vi "FPGA 796xR - Bak20470818.vi"() -> ()   [LabVIEW 2015]
uses:
  Controls/FPGA_Frame State.ctl
  <vilib>/Platform/TimedLoop/XDataNode/timing_clust.ctl
  <vilib>/Platform/TimedLoop/XDataNode/nitl_modes.ctl
  <vilib>/Platform/TimedLoop/XDataNode/wakeup.ctl
  <vilib>/rvi/Emulation/niFpgaSctlEmulationGetInTimedLoop.vi
  <vilib>/rvi/Emulation/niFpgaProcessEmulError.vi
  <vilib>/rvi/Emulation/niFpgaEmulationReportErrorSimple.vi
  <vilib>/rvi/Emulation/niFpgaGetClockAttributes.vi
  <vilib>/rvi/Emulation/niFpgaCriticalErrorInLSC.vi
  <vilib>/rvi/eio/common/nirviEmuTemplateMethod_errors.vi
  <vilib>/rvi/interface/RandomDataEmulation/niFpgaRandomDataHandleErrors.vi
  <vilib>/rvi/Memory/Memory_Emulation/nirvimemoryFastEmulation.vi
  <vilib>/rvi/Memory/Memory_Emulation/nirvimemoryEmulation.vi
  <vilib>/rvi/Emulation/niFpgaEmulationIsFPGAContextNoSignature.vi
  <vilib>/rvi/DataTransferAndStorage/Container/Common/niFpgaContainerGetUniqueNameForEmu.vi
  <vilib>/rvi/errors/nirviReportUnexpectedCaseInternalError (U32).vi
  <vilib>/Platform/TimedLoop/XDataNode/XDataNode.xnode
  <vilib>/eio/EIONode/EIONode.xnode
  <vilib>/rvi/DataTransferAndStorage/Container/XNode/niFpgaContainer.xnode
  <vilib>/rvi/interface/RandomDataEmulation/nirviRandomDataFpgaReadWriteTemplate.vi
  <vilib>/rvi/FXPMathLib/FxpMul/XNode/nifxpmath_Multiplier.xnode
  <vilib>/rvi/FXPMathLib/FxpAdd/XNode/nifxpmath_Add.xnode
  <vilib>/Platform/TimedLoop/XDataNode/XDNodeRunTimeDep.lvlib
  <instrlib>/_niInstr/Basic Elements/v1/FPGA/niInstr Basic Elements v1 FPGA.lvlib
  <vilib>/rvi/FXPMathLib/sim/FxpSim.dll
panel:
  out "Acq. Point Dis.":u16
  in  "Acq.Start":u16
  in  "Acq.Start FXP":fxp<+,16,0>
  out "Acq Pixel Number":u32
  out "AcqPoint 元素数量":u32
  in  "Microscope":enum16{"Miniature", "Benchtop"}(ring)
  out "No Remind":bool
  out "Remind Element":u32
  in  "FOCUS":bool
  out "Wait Frame State":T1
  in  "Line":u16
  in  "Pixel/Line":u16
  out "Adapter Module Present":bool
  out "Adapter Module ID Expected":u32
  out "Adapter Module ID Inserted":u32
  out "Adapter Module Initialization Done":bool
  out "Adapter Module ID Mismatch":bool
  in  "Adapter Module Do User Command Commit":bool caption="(Mech Action: Latch)"
  in  "Adapter Module User Command":u8
  out "Adapter Module User Command Idle":bool
  out "Adapter Module User Command Status":u8
  in  "Adapter Module User Data 0":u8
  in  "Adapter Module User Data 1":u8
  out "Adapter Module PLL Locked":bool
  # "Acquisition Parameters"
  # "Acquisition Control"
  # "User Command Load"
  # "Fpga status"
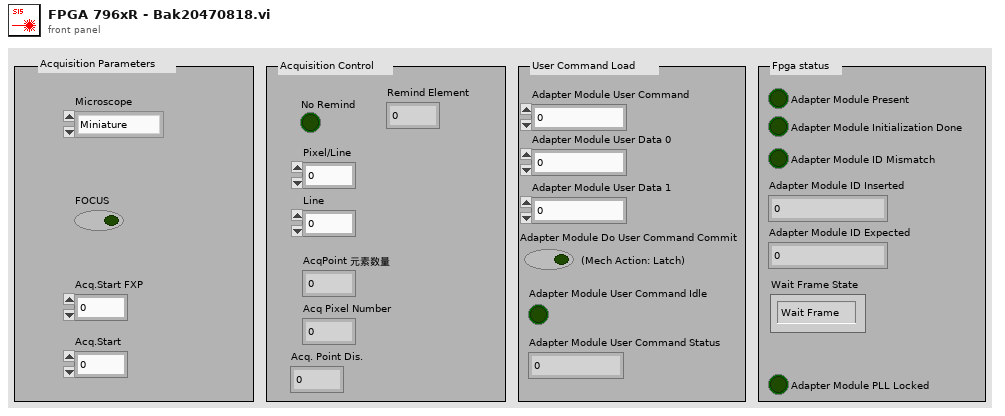
[diagram p1: front panel]
types:
  T1 = typedef "FPGA_Frame State.ctl" = enum16{"Wait Frame", "Start Frame", "Framing"}
  T2 = typedef "XDNodeRunTimeDep.lvlib/timing_clust.ctl" = cluster{"Expected End [f-1]":u64, "Actual End [f-1]":u64, "Finished Late? [f-1]":bool, "Expected End [i-1]":u64, "Actual End [i-1]":u64, "Finished Late? [i-1]":bool, "Expected Start [i]":u64, "Actual Start [i]":u64, "Expected Start [f]":u64, "Actual Start [f]":u64, "Source Name":string, "Structure Name":string, "Period":i64, "Deadline":i64, "Offset":i64, "Start":i64, "Priority":i32, "Timeout":i32, "Mode":T3, "Wakeup Reason":T4, "Error":errorcluster, "Source Type":string, "Secondary Source Type":string, "Global End Time":u64, "Global Start Time":u64, "Frame Duration":u64, "Iteration Duration":u64, "Assigned CPU":i32, "I/O Scan Engine Mode":u32}
  T3 = typedef "XDNodeRunTimeDep.lvlib/nitl_modes.ctl" = enum32{"No Change", "Process missed periods, maintain original phase", "Discard missed periods, maintain original phase", "Process missed periods, ignore original phase", "Discard missed periods, ignore original phase"}
  T4 = typedef "XDNodeRunTimeDep.lvlib/wakeup.ctl" = enum32{"Normal", "Aborted", "Asynchronous wakeup", "Timing source error", "Timed loop error", "Timeout"}
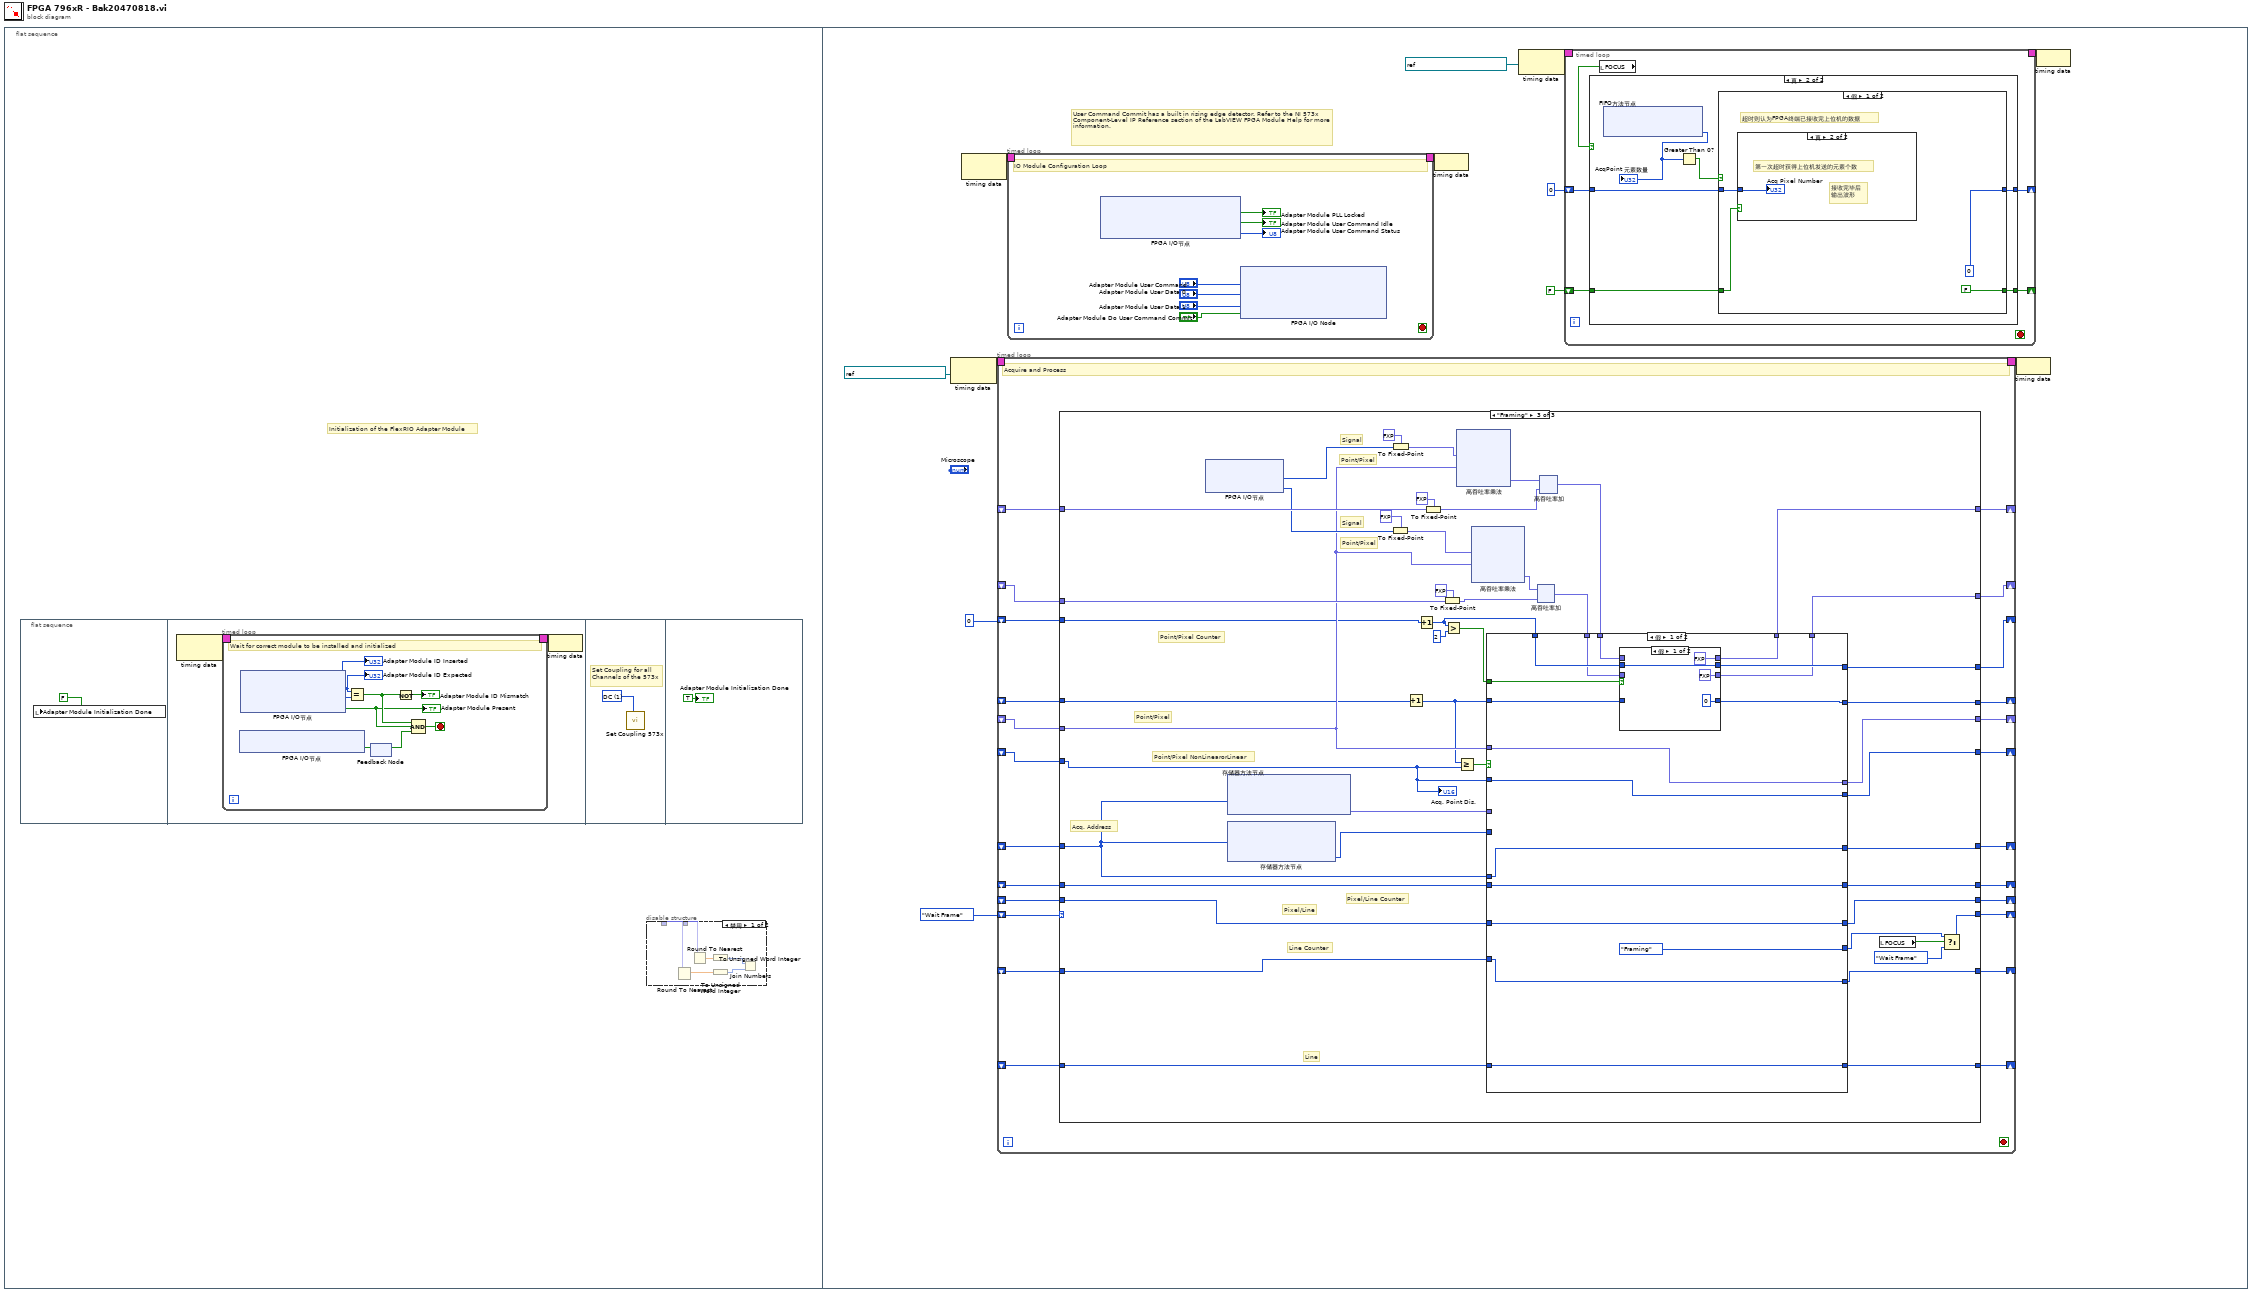
[diagram p0: block diagram]
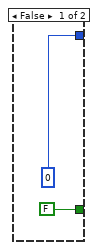
[diagram p3: hidden frame]
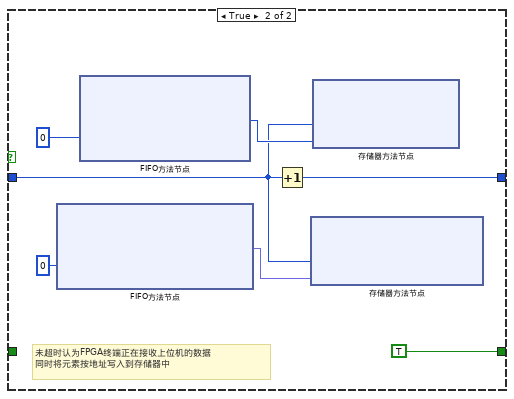
[diagram p5: hidden frame]
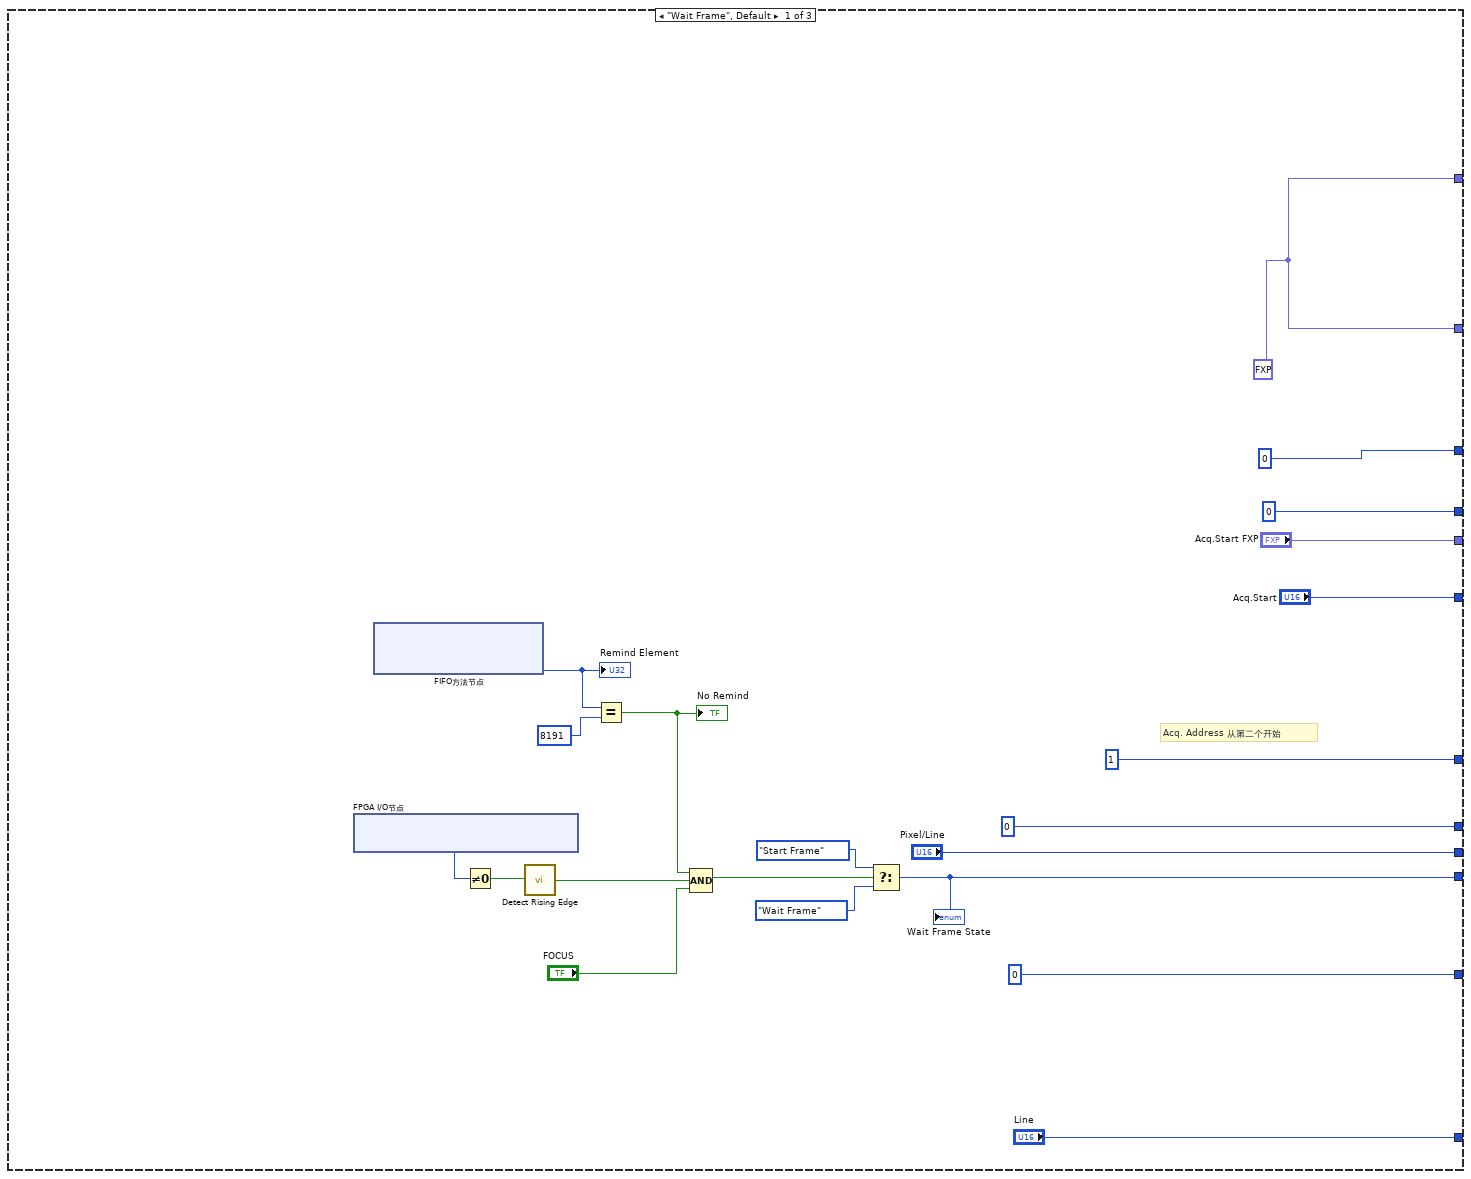
[diagram p6: hidden frame]
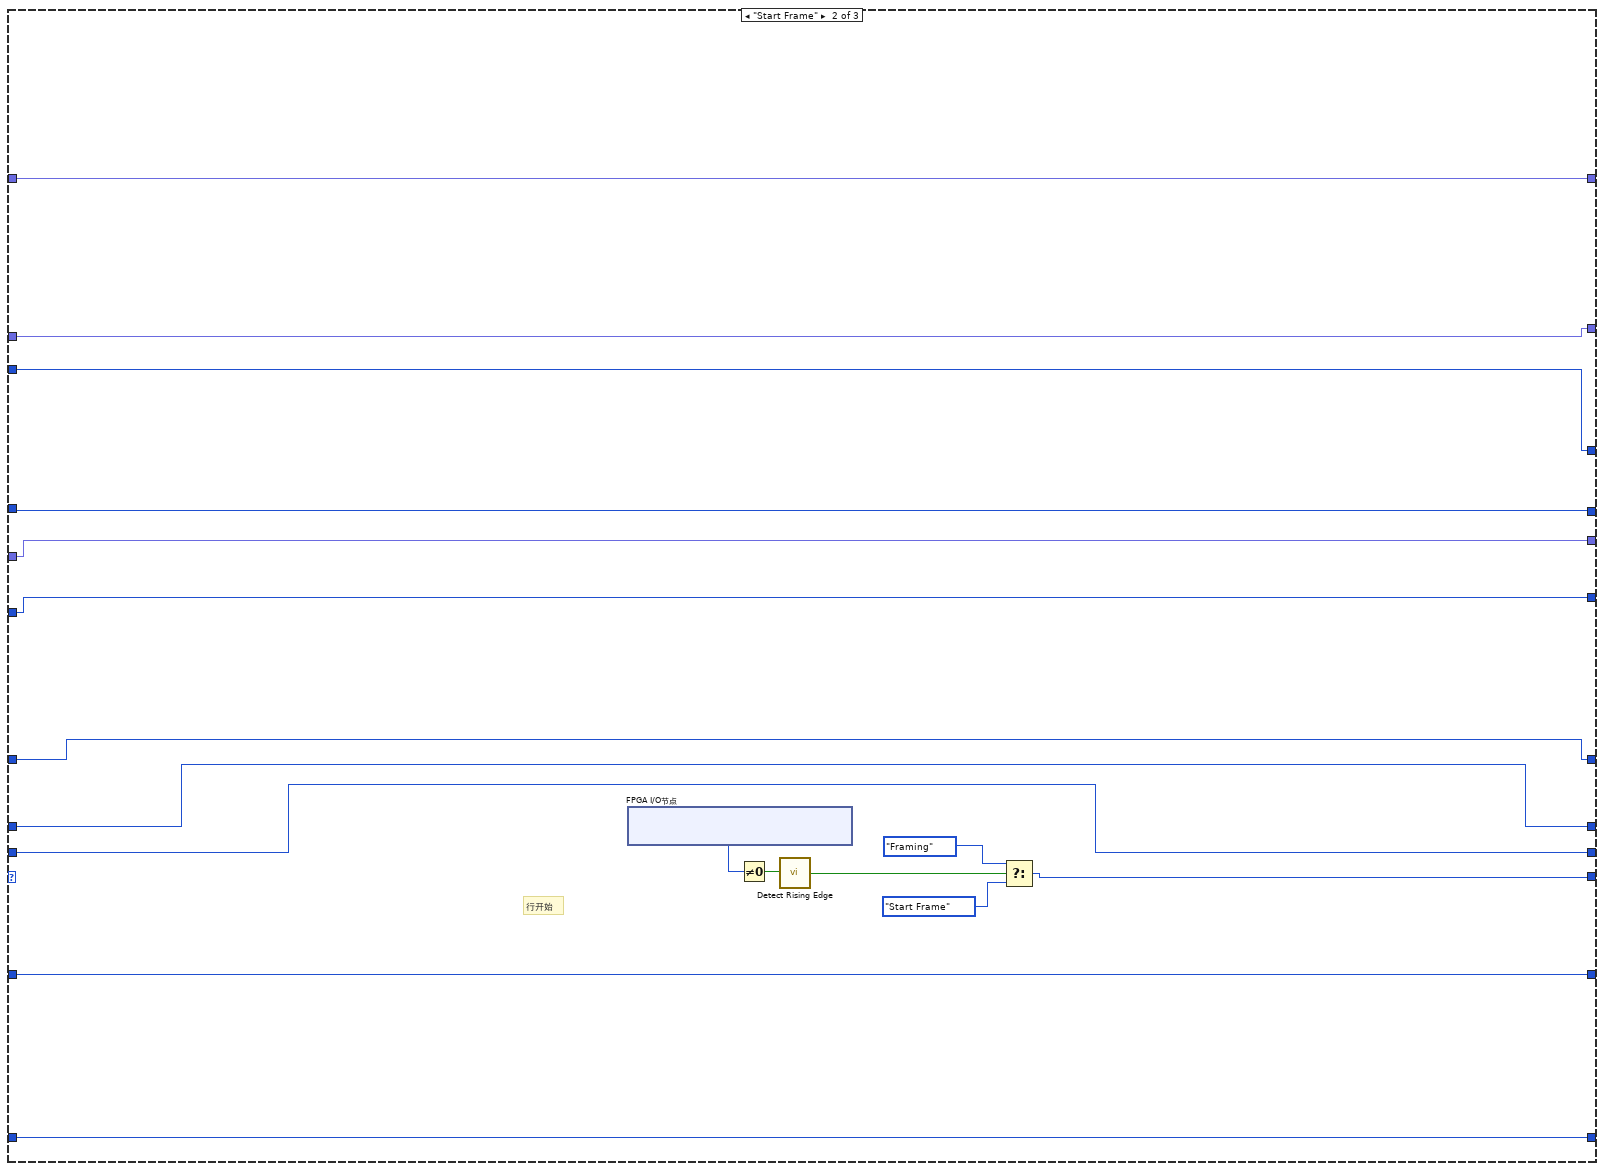
[diagram p7: hidden frame]
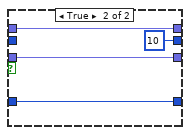
[diagram p8: hidden frame]
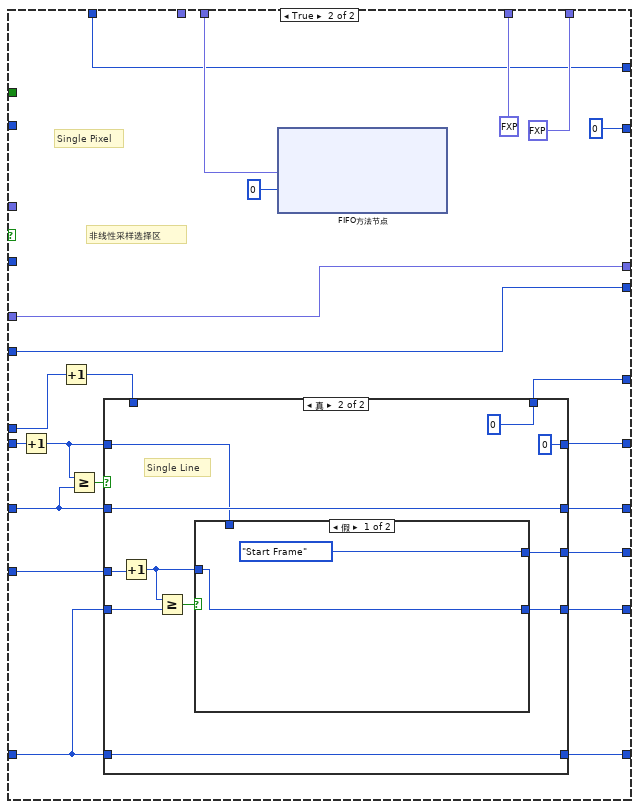
[diagram p9: hidden frame]
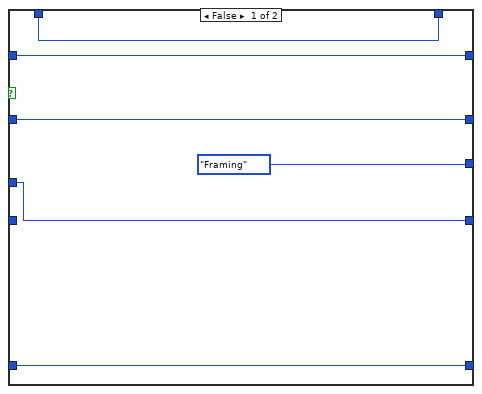
[diagram p10: hidden frame]
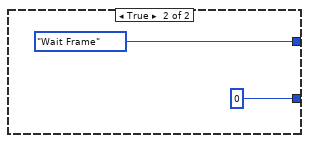
[diagram p11: hidden frame]
diagram:
  n1 = flat-sequence {
    frame #0 {
      # "Initialization of the FlexRIO Adapter Module"
      n2 = flat-sequence {
        frame #0 {
          n3 = local write "Adapter Module Initialization Done"(FALSE ("InitializationDone")) -> ()
        }
        frame #1 {
          n4 = node-c288() -> (w9:T2)  [unwired: 1 in]
          n5 = timed-loop {
            timing: w9 -> [_]
            timing-out: [_] -> w8
            stop <- w16 stop-if-true
            # "Wait for correct module to be installed and initialized"
            n6 = xnode "FPGA I/O节点"() -> ("IO Module\\Initialization Done"=w11:bool)  [unwired: 1 in, 1 out]
            n7 = xnode "FPGA I/O节点"() -> ("Expected IO Module ID"=w17:u32, "Inserted IO Module ID"=w15:u32, "IO Module Present"=w12:bool)  [unwired: 3 in, 3 out]
            "Adapter Module ID Inserted" <- w15
            "Adapter Module ID Expected" <- w17
            "Adapter Module Present" <- w12
            n8 = Equal?(x=w17, y=w15) -> (x = y?=w13:bool)
            n9 = feedback-in #1(w11) -> ()
            n10 = feedback #1() -> (w10:bool)  [unwired: 1 in]
            n11 = Not(x=w13) -> (.not. x?=→"Adapter Module ID Mismatch":bool)
            n12 = Compound Arithmetic op=AND(w13, w12, w10) -> (w16:bool)
          }
          n13 = node-c288(w8) -> ()
        }
        frame #2 {
          w22 = u8 1 items=["DC"=1, "AC"=0] ("Coupling")
          # "Set Coupling for all\nChannels of the 573x"
          n14 = call "Set Coupling 573x.vi"("Coupling"=w22) -> ()  [unwired: 11 in]
        }
        frame #3 {
          "Adapter Module Initialization Done" <- TRUE ("InitializationDone")
        }
      }
      n15 = disable-structure shown="禁用" {
        disable-tunnel: _ -> [w6 _]
        disable-tunnel: _ -> [w4 _]
        frame Disabled {
          n16 = Round To Nearest(number=w4) -> (nearest integer value=w2:dbl)
          n17 = Round To Nearest(number=w6) -> (nearest integer value=w5:dbl)
          n18 = To Unsigned Word Integer(number=w5) -> (unsigned 16bit integer=w3:u16)
          n19 = To Unsigned Word Integer(number=w2) -> (unsigned 16bit integer=w1:u16)
          n20 = Join Numbers(hi=w3, lo=w1) -> ()  [unwired: 1 out]
        }
        frame Enabled {
        }
      }
    }
    frame #1 {
      # "User Command Commit has a built in rising edge detector. Refer to the NI 573x Component-Level IP Reference section of the LabVIEW FPGA Module Help for more information."
      n21 = node-c288(refnum<k21> "IO Module\\Sample Clock" ("Source Name")) -> (w33:T2)
      n22 = node-c288() -> (w35:T2)  [unwired: 1 in]
      n23 = timed-loop {
        timing: w33 -> [_]
        timing-out: [_] -> w32
        shift-right: [w89] -> _
        shift-left: FPGA_Frame_State."Wait Frame" ("Line State") -> [w90]
        shift-right: [w87] -> _
        shift-left: _ -> [w88]
        shift-right: [w85] -> _
        shift-left: _ -> [w86]
        shift-right: [w83] -> _
        shift-left: _ -> [w84]
        shift-right: [w81] -> _
        shift-left: _ -> [w82]
        shift-right: [w79] -> _
        shift-left: _ -> [w80]
        shift-right: [w77] -> _
        shift-left: _ -> [w78]
        shift-right: [w75] -> _
        shift-left: _ -> [w76]
        shift-right: [w73] -> _
        shift-left: _ -> [w74]
        shift-right: [w71] -> _
        shift-left: _ -> [w72]
        shift-right: [w70] -> _
        shift-left: _ -> [w69]
        shift-right: [w67] -> _
        shift-left: u8 0 ("超时") -> [w68]
        stop <- _ stop-if-true
        # "Acquire and Process"
        n24 = case shown="\"Framing\"" w90 {
          tunnel: [w107 w124 w175] -> w89
          tunnel: w88 -> [_ w116 w134]
          tunnel: [u16 0 ("t") w116 w174] -> w87
          tunnel: w86 -> [_ w118 w173]
          tunnel: [u16 0 ("t") w118 w172] -> w85
          tunnel: w84 -> [_ w117 w171]
          tunnel: [w95 w117 w170] -> w83
          tunnel: w82 -> [_ w126 w169]
          tunnel: [u16 0 ("t") w126 w168] -> w81
          tunnel: w80 -> [_ w121 w142]
          tunnel: ["Acq.Start FXP" w121 w152] -> w79
          tunnel: w78 -> [_ w120 w167]
          tunnel: ["Pixel/Line" w120 w166] -> w77
          tunnel: w76 -> [_ w119 w165]
          tunnel: ["Line" w119 w164] -> w75
          tunnel: w74 -> [_ w115 w154]
          tunnel: [w95 w115 w153] -> w73
          tunnel: w72 -> [_ w114 w138]
          tunnel: ["Acq.Start" w114 w144] -> w71
          tunnel: [u32 1 ("地址") w113 w143] -> w70
          tunnel: w69 -> [_ w113 w139]
          tunnel: w68 -> [_ w112 w133]
          tunnel: [u8 0 ("超时") w112 w130] -> w67
          frame "Wait Frame", Default {
            w95 = fxp<+,32,16> 0.0 ("x")
            # "Acq. Address 从第二个开始"
            n25 = xnode "FPGA I/O节点"() -> ("IO Module\\DIO Port 1 Rd Data"=w109:u8)  [unwired: 1 in, 1 out]
            n26 = xnode ("FIFO方法节点")() -> ("待写入元素数量"=w101:u32)  [unwired: 1 in, 1 out]
            "Remind Element" <- w101
            n27 = Not Equal To 0?(x=w109) -> (x != 0?=w110:bool)
            n28 = call <instrlib>:"Detect Rising Edge.vi"("signal"=w110) -> ("edge detected"=w96:bool)  [unwired: 14 in]
            n29 = Equal?(x=w101, y=u32 8191) -> (x = y?=w98:bool)
            "No Remind" <- w98
            n30 = Compound Arithmetic op=AND(w98, w96, "FOCUS") -> (w97:bool)
            n31 = Select(t=FPGA_Frame_State."Start Frame" ("Line State"), s=w97, f=FPGA_Frame_State."Wait Frame" ("Line State")) -> (s? t:f=w107:T1)
            "Wait Frame State" <- w107
          }
          frame "Start Frame" {
            # "行开始"
            n32 = xnode "FPGA I/O节点"() -> ("IO Module\\DIO Port 0 Rd Data"=w127:u8)  [unwired: 1 in, 1 out]
            n33 = Not Equal To 0?(x=w127) -> (x != 0?=w128:bool)
            n34 = call <instrlib>:"Detect Rising Edge.vi"("signal"=w128) -> ("edge detected"=w125:bool)  [unwired: 14 in]
            n35 = Select(t=FPGA_Frame_State."Framing" ("Line State"), s=w125, f=FPGA_Frame_State."Start Frame" ("Line State")) -> (s? t:f=w124:T1)
          }
          frame "Framing" {
            # "Acq. Address"
            # "Pixel/Line Counter"
            # "Point/Pixel NonLinearorLinear"
            # "Signal"
            # "Signal"
            # "Point/Pixel"
            # "Point/Pixel"
            # "Line Counter"
            # "Line"
            # "Point/Pixel Counter"
            # "Pixel/Line"
            # "Point/Pixel"
            n36 = xnode "FPGA I/O节点"() -> ("IO Module\\AI 0"=w162:u16, "IO Module\\AI 1"=w156:u16)  [unwired: 2 in, 2 out]
            n37 = xnode ("存储器方法节点")("地址"=w139) -> ("数据"=w140:fxp<+,16,0>)  [unwired: 1 in, 1 out]
            n38 = xnode ("存储器方法节点")("地址"=w139) -> ("数据"=w141:u16)  [unwired: 1 in, 1 out]
            n39 = To Fixed-Point(fixed-point type=fxp<+,18,16> 0.0 ("x"), number=w156) -> (fixed-point=w151:fxp<+,18,16>)
            n40 = To Fixed-Point(fixed-point type=fxp<+,18,16> 0.0 ("x"), number=w162) -> (fixed-point=w150:fxp<+,18,16>)
            n41 = Increment(x=w134) -> (x+1=w137:u16)
            n42 = Increment(x=w133) -> (x+1=w129:u8)
            n43 = To Fixed-Point(fixed-point type=fxp<+,32,16> 0.0 ("x"), number=w171) -> (fixed-point=w147:fxp<+,32,16>)
            n44 = To Fixed-Point(fixed-point type=fxp<+,32,16> 0.0 ("x"), number=w154) -> (fixed-point=w145:fxp<+,32,16>)
            n45 = Greater?(x=w129, y=u8 2 ("超时")) -> (0:w131:bool)
            n46 = xnode ("高吞吐率乘法")("x"=w150, "y"=w142) -> ("x*y"=w148:fxp<+,32,16>)
            n47 = Greater Or Equal?(x=w137, y=w138) -> (x >= y?=w160:bool)
            n48 = xnode ("高吞吐率乘法")("x"=w151, "y"=w142) -> ("x*y"=w146:fxp<+,32,16>)
            n49 = xnode ("高吞吐率加")("x"=w146, "y"=w145) -> ("x+y"=w135:fxp<+,33,17>)
            n50 = xnode ("高吞吐率加")("x"=w148, "y"=w147) -> ("x+y"=w136:fxp<+,33,17>)
            n51 = case shown="假" w160 {
              tunnel: w136 -> [w180 w207]
              tunnel: [w181 fxp<+,32,16> 0.0 ("x")] -> w170
              tunnel: [w177 u16 0 ("t")] -> w174
              tunnel: w137 -> [w176 _]
              tunnel: w173 -> [w189 w214]
              tunnel: w169 -> [w188 w220]
              tunnel: [w188 w219] -> w168
              tunnel: [FPGA_Frame_State."Framing" ("Line State") w218] -> w158
              tunnel: [w189 w213] -> w172
              tunnel: w165 -> [w191 w216]
              tunnel: [w190 w215] -> w166
              tunnel: w167 -> [w190 w209]
              tunnel: [w191 w217] -> w164
              tunnel: w135 -> [w178 _]
              tunnel: [w179 fxp<+,32,16> 0.0 ("x")] -> w153
              tunnel: w142 -> [w187 _]
              tunnel: [w187 w204] -> w152
              tunnel: w138 -> [w186 _]
              tunnel: [w186 w203] -> w144
              tunnel: w141 -> [_ w203]
              tunnel: [w185 w205] -> w143
              tunnel: w140 -> [_ w204]
              tunnel: w139 -> [w185 w202]
              tunnel: w131 -> [w184 _]
              tunnel: [w183 w201] -> w130
              tunnel: w129 -> [w182 w201]
              frame False {
                n52 = case shown="假" w184 {
                  tunnel: [w194 u8 10] -> w183
                  tunnel: w182 -> [w194 _]
                  tunnel: [fxp<+,33,17> 0.0 ("x+y") w200] -> w181
                  tunnel: w180 -> [_ w200]
                  tunnel: [fxp<+,33,17> 0.0 ("x+y") w199] -> w179
                  tunnel: w178 -> [_ w199]
                  tunnel: [u16 0 w197] -> w177
                  tunnel: w176 -> [_ w197]
                  frame False {
                  }
                  frame True {
                  }
                }
              }
              frame True {
                # "Single Pixel"
                # "非线性采样选择区"
                n53 = Increment(x=w214) -> (x+1=w208:u16)
                n54 = Increment(x=w202) -> (x+1=w206:u32)
                n55 = Greater Or Equal?(x=w208, y=w209) -> (x >= y?=w212:bool)
                n56 = case shown="真" w212 {
                  tunnel: w220 -> [w224 w239]
                  tunnel: [w224 w238] -> w219
                  tunnel: [FPGA_Frame_State."Framing" ("Line State") w237] -> w218
                  tunnel: w216 -> [_ w234]
                  tunnel: [w228 w233] -> w217
                  tunnel: w216 -> [w228 w233]
                  tunnel: [w227 w232] -> w215
                  tunnel: w209 -> [w227 w232]
                  tunnel: [w226 u16 0] -> w213
                  tunnel: w208 -> [w226 w230]
                  tunnel: w206 -> [w223 _]
                  tunnel: [w223 u32 0] -> w205
                  frame False {
                  }
                  frame True {
                    # "Single Line"
                    n57 = Increment(x=w239) -> (x+1=w235:u16)
                    n58 = Greater Or Equal?(x=w235, y=w234) -> (x >= y?=w236:bool)
                    n59 = case shown="假" w236 {
                      tunnel: w235 -> [w240 _]
                      tunnel: [w240 u16 0] -> w238
                      tunnel: [FPGA_Frame_State."Start Frame" ("Line State") FPGA_Frame_State."Wait Frame" ("Line State")] -> w237
                      tunnel: w230 -> [_ _]
                      frame False {
                      }
                      frame True {
                      }
                    }
                  }
                }
                n60 = xnode ("FIFO方法节点")("元素"=w207, "超时"=0) -> ()  [unwired: 1 in, 2 out]
              }
            }
            n61 = local read "FOCUS"() -> (w159:bool)
            n62 = Select(t=w158, s=w159, f=FPGA_Frame_State."Wait Frame" ("Line State")) -> (s? t:f=w175:T1)
            "Acq. Point Dis." <- w138
          }
        }
      }
      n63 = timed-loop {
        timing: w35 -> [_]
        timing-out: [_] -> w34
        stop <- _ stop-if-true
        # "IO Module Configuration Loop"
        n64 = xnode "FPGA I/O节点"() -> ("IO Module\\PLL Locked"=→"Adapter Module PLL Locked":bool, "IO Module\\User Command Idle"=→"Adapter Module User Command Idle":bool, "IO Module\\User Command Status"=→"Adapter Module User Command Status":u8)  [unwired: 3 in, 3 out]
        n65 = xnode ("FPGA I/O Node")("IO Module\\User Command"="Adapter Module User Command", "IO Module\\User Data 0"="Adapter Module User Data 0", "IO Module\\User Data 1"="Adapter Module User Data 1", "IO Module\\User Command Commit"="Adapter Module Do User Command Commit") -> ()  [unwired: 4 in, 4 out]
      }
      n66 = node-c288(w34) -> ()
      n67 = node-c288(refnum<k21> "IO Module\\Sample Clock" ("Source Name")) -> (w29:T2)
      n68 = timed-loop {
        shift-right: [w39] -> _
        shift-left: u32 0 ("地址") -> [w40]
        shift-right: [w37] -> _
        shift-left: FALSE ("执行") -> [w38]
        timing: w29 -> [_]
        timing-out: [_] -> w28
        stop <- _ stop-if-true
        n69 = local read "FOCUS"() -> (w36:bool)
        n70 = case shown="真" w36 {
          tunnel: w40 -> [_ w48]
          tunnel: [u32 0 w47] -> w39
          tunnel: w38 -> [_ w46]
          tunnel: [FALSE w45] -> w37
          frame False {
          }
          frame True {
            n71 = xnode ("FIFO方法节点")() -> ("待读取元素数量"=w43:u32)  [unwired: 1 in, 1 out]
            "AcqPoint 元素数量" <- w43
            n72 = Greater Than 0?(x=w43) -> (x > 0?=w44:bool)
            n73 = case shown="假" w44 {
              tunnel: w48 -> [w50 w54]
              tunnel: [u32 0 w59] -> w47
              tunnel: w46 -> [w51 _]
              tunnel: [FALSE TRUE] -> w45
              frame False {
                # "超时则认为FPGA终端已接收完上位机的数据"
                n74 = case shown="真" w51 {
                  tunnel: w50 -> [_ w53]
                  frame False {
                  }
                  frame True {
                    # "接收完毕后\n输出波形"
                    # "第一次超时获得上位机发送的元素个数"
                    "Acq Pixel Number" <- w53
                  }
                }
              }
              frame True {
                # "未超时认为FPGA终端正在接收上位机的数据\n同时将元素按地址写入到存储器中"
                n75 = xnode ("FIFO方法节点")("超时"=0) -> ("元素"=w56:fxp<+,16,0>)  [unwired: 1 in, 2 out]
                n76 = xnode ("FIFO方法节点")("超时"=0) -> ("元素"=w57:u16)  [unwired: 1 in, 2 out]
                n77 = Increment(x=w54) -> (x+1=w59:u32)
                n78 = xnode ("存储器方法节点")("地址"=w54, "数据"=w56) -> ()  [unwired: 1 in, 1 out]
                n79 = xnode ("存储器方法节点")("地址"=w54, "数据"=w57) -> ()  [unwired: 1 in, 1 out]
              }
            }
          }
        }
      }
      n80 = node-c288(w32) -> ()
      n81 = node-c288(w28) -> ()
    }
  }
